vi "Out_S7F28.vi"(8 "error in (no error)":errorcluster, 11 "S7 Message Class in":refnum<class "S7 Message Class.lvclass">) -> (0 "error out":errorcluster, 3 "S7 Message Class out":refnum<class "S7 Message Class.lvclass">)   [LabVIEW 2020, in "SECS Communication.lvlib" / "S7 Message Class.lvclass"]
uses:
  S7 Message Class.lvclass
  D:/Dropbox/SECS/LabVIEW Code/Com/SECS Communication/SECS-II Class/SECS-II Class.lvclass
  S7 Message Class.lvclass/S7 Message Class.ctl
  SECS-II Class/SECS-II Class.lvclass
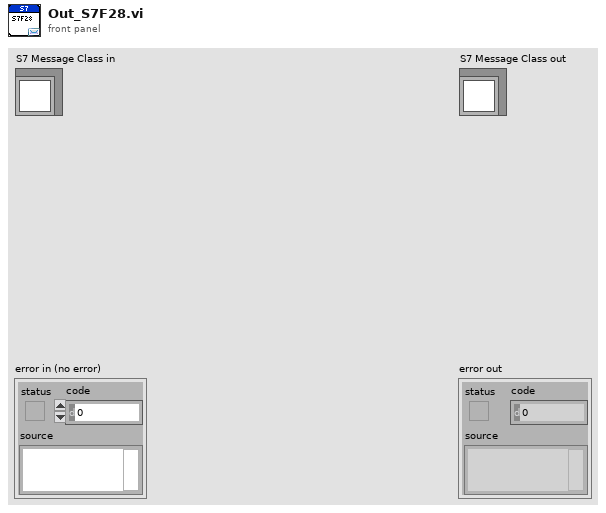
[diagram p1: front panel]
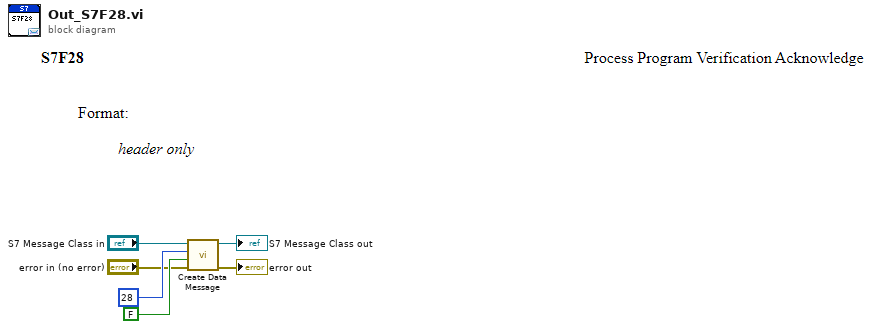
[diagram p0: block diagram]
diagram:
  n1 = call "Create Data Message.vi"("error in (no error)"="error in (no error)", "W-Bit"=FALSE, "Function"=u8 28, "SECS-II Class in"="S7 Message Class in") -> ("error out"=→"error out":errorcluster, "SECS-II Class out"=→"S7 Message Class out":refnum<class "S7 Message Class.lvclass">)  [unwired: 6 in]
